vi "Close.vi"(8 "error in (no error)":errorcluster, 11 "DataShare in":refnum<class "DataShare.lvclass">) -> (0 "error out":errorcluster, 3 "DataShare out":refnum<class "DataShare.lvclass">)   [LabVIEW 2014, in "DataShare.lvclass"]
uses:
  DataShare.lvclass
  DataShare.lvclass/DataShare.ctl
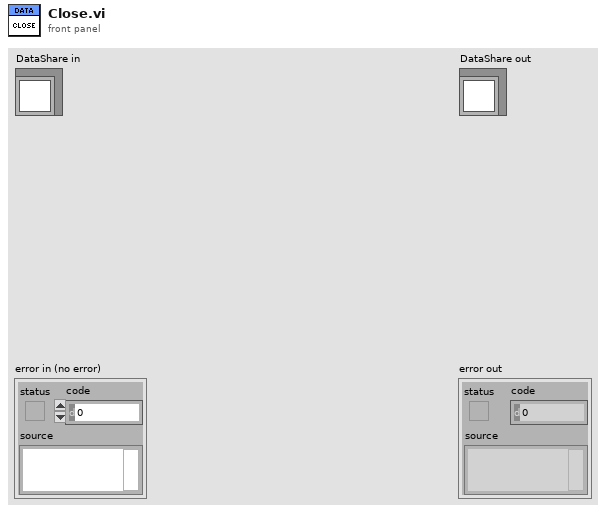
[diagram p1: front panel]
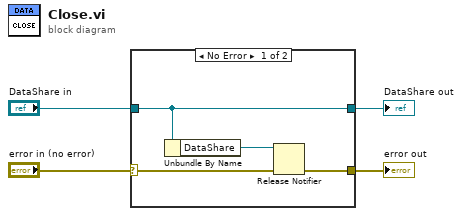
[diagram p0: block diagram]
diagram:
  n1 = case shown="No Error" "error in (no error)" {
    selector: "error in (no error)" -> [w6 w10]
    tunnel: [w5 w10] -> w3
    tunnel: [w8 w9] -> w1
    tunnel: "DataShare in" -> [w8 w9]
    frame No Error {
      n2 = Unbundle By Name(w8) -> ("DataShare"=w7:refnum<notifier>)
      n3 = Release Notifier(notifier=w7, error in (no error)=w6) -> (error out=w5:errorcluster)  [unwired: 1 in, 2 out]
    }
    frame Error {
    }
  }
  "error out" <- w3
  "DataShare out" <- w1
